vi "Lvi Trigger Settings.vi"(0 "TaskRef":i32, 1 "SetPreTrigger":bool, 5 "TriggerSource":u32, 7 "PreTriggerSource":u32, 9 "SetTrigger":bool, 11 "error in (no error)":errorcluster) -> (4 "TaskRef out":i32, 6 "TriggerSource out":u32, 8 "PreTriggerSource out":u32, 10 "function return":u32(ring), 15 "error out":errorcluster)   [LabVIEW 2022 SP3, in "DtLvLink.lvlib"]
doc: "Calls directly into the entry points of the DLL of the Data Acq SDK to set trigger properties and return information about the trigger source of the device. This VI is used by the higher-level VI, DtOLTriggerSource."
uses:
  DtLvLink.lvlib
  <userlib>/LV-Link3/DtLvLink_64.dll
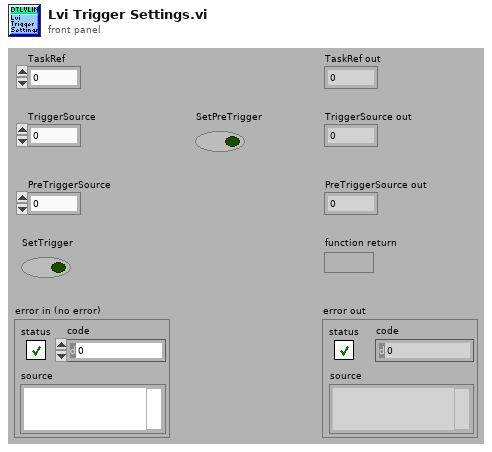
[diagram p1: front panel]
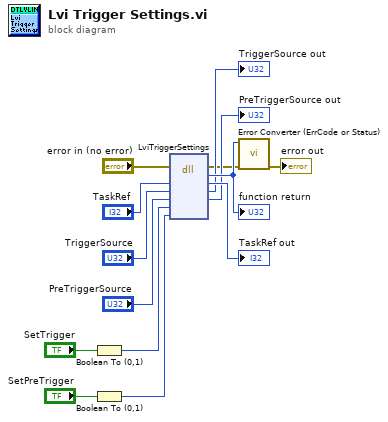
[diagram p0: block diagram]
diagram:
  n1 = Boolean To (0,1)(Boolean="SetTrigger") -> (0, 1=w6:i16)
  n2 = Boolean To (0,1)(Boolean="SetPreTrigger") -> (0, 1=w4:i16)
  n3 = dll-call lib="C:/Program Files/National Instruments/LabVIEW 2022/user.lib/LV-Link3/DtLvLink_64.*" fn="LviTriggerSettings"(error in="error in (no error)", "TaskRef"="TaskRef", "TriggerSource"="TriggerSource", "PreTriggerSource"="PreTriggerSource", "SetTrigger"=w6, "SetPreTrigger"=w4) -> (error out=w2:errorcluster, w14:u32, "TaskRef"=→"TaskRef out":i32, "TriggerSource"=→"TriggerSource out":u32, "PreTriggerSource"=→"PreTriggerSource out":u32)  [unwired: 4 in, 1 out]
  "function return" <- w14
  n4 = call "Error Converter (ErrCode or Status).vi"("error in (no error)"=w2, "error code"=w14) -> ("error out"=→"error out":errorcluster)  [unwired: 9 in]
